vi "Destroyer UserEvent.vi"(8 "error in (no error)":errorcluster, 11 "Guardar Tipo CSV in":refnum<class "Guardar Tipo CSV.lvclass">) -> (0 "error out":errorcluster, 3 "Guardar Tipo CSV out":refnum<class "Guardar Tipo CSV.lvclass">)   [LabVIEW 2020, in "Guardar Tipo CSV.lvlib" / "Guardar Tipo CSV.lvclass"]
uses:
  Guardar Tipo CSV.lvclass
  Guardar Tipo CSV.lvclass/Guardar Tipo CSV.ctl
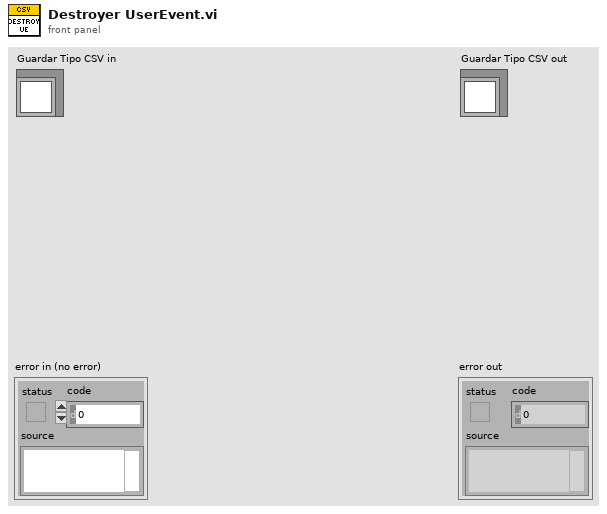
[diagram p1: front panel]
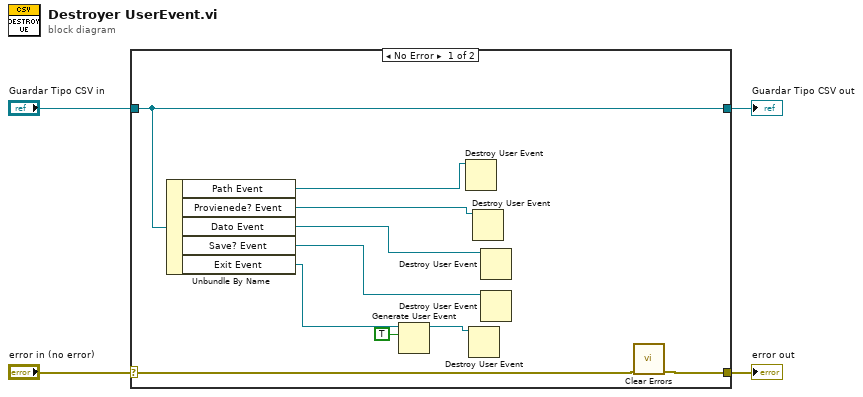
[diagram p0: block diagram]
diagram:
  n1 = case shown="No Error" "error in (no error)" {
    selector: "error in (no error)" -> [w6 w16]
    tunnel: [w5 w16] -> w3
    tunnel: [w14 w15] -> w1
    tunnel: "Guardar Tipo CSV in" -> [w14 w15]
    frame No Error {
      n2 = Unbundle By Name(w14) -> ("Path Event"=w13:refnum<user-event>, "Provienede? Event"=w12:refnum<user-event>, "Dato Event"=w11:refnum<user-event>, "Save? Event"=w10:refnum<user-event>, "Exit Event"=w9:refnum<user-event>)
      n3 = Generate User Event(user event=w9, event data cluster=TRUE ("event data")) -> (user event out=w7:refnum<user-event>)  [unwired: 2 in, 1 out]
      n4 = Destroy User Event(user event=w13) -> ()  [unwired: 1 in, 1 out]
      n5 = Destroy User Event(user event=w7) -> ()  [unwired: 1 in, 1 out]
      n6 = Destroy User Event(user event=w12) -> ()  [unwired: 1 in, 1 out]
      n7 = Destroy User Event(user event=w11) -> ()  [unwired: 1 in, 1 out]
      n8 = Destroy User Event(user event=w10) -> ()  [unwired: 1 in, 1 out]
      n9 = call <vilib>:"Clear Errors.vi"("error in (no error)"=w6) -> ("error out"=w5:errorcluster)  [unwired: 5 in, 1 out]
    }
    frame Error {
    }
  }
  "error out" <- w3
  "Guardar Tipo CSV out" <- w1
